vi "B7_72.vi"(4 "error in":T13, 7 "Command":T14) -> (0 "error out":T13, 3 "Response":T11)   [LabVIEW 2018]
uses:
  MOKO_LabViewLibrary/MokoLowLevel/MokoLowLovelControl/MLLC_Command.ctl
  MOKO_LabViewLibrary/MokoLowLevel/MokoLowLovelControl/MLLC_Error.ctl
  MOKO_LabViewLibrary/MokoLowLevel/MokoLowLovelControl/MLLC_Mode.ctl
  MOKO_LabViewLibrary/MokoLowLevel/MokoLowLovelControl/MLLC_Response.ctl
  MOKO_LabViewLibrary/MokoLowLevel/MokoLowLovelControl/MLLC_DriverName.ctl
  MOKO_LabViewLibrary/MokoLowLevel/MokoLowLovelControl/MLLC_ResponseInit.ctl
  MOKO_LabViewLibrary/MokoLowLevel/MokoLowLovelControl/MLLC_Request.ctl
  MOKO_LabViewLibrary/MokoLowLevel/MokoLowLovelControl/MLLC_ErrorCode.ctl
  MOKO_LabViewLibrary/MokoLowLevel/MokoLowLovelControl/MLLC_ConnectCluster.ctl
  MOKO_LabViewLibrary/MokoLowLevel/MokoLowLovelControl/MLLC_InterfaceType.ctl
  MOKO_LabViewLibrary/MokoLowLevel/MokoLowLovelControl/MLLC_OpenedSession.ctl
  MOKO_LabViewLibrary/MokoLowLevel/MokoLowLovelControl/MLLC_InterfaceSettings.ctl
  MOKO_LabViewLibrary/MokoLowLevel/MokoLowLovelControl/MLLC_InterfaceKind.ctl
  MOKO_LabViewLibrary/MokoLowLevel/MokoLowLovelControl/MLLC_Rs232Settings.ctl
panel:
  in  "Settings":T7={"Data"={"Connect"={"InterfaceType"=enum."VISA", "OpenedSession"="COM1", "InterfaceSettings"={"Interface"=enum."RS232", "EOS 4 read"=enum."LF (\\n)", "EOS 4 write"=enum."LF (\\n)", "TMO, ms"=10000, "Sett"=variant(cluster{"Baud Rate":u32, "Data Bits":u16, "Parity":u16, "Stop Bits":u16, "Flow Control":u16, "Eho":bool} {"Baud Rate"=75, "Data Bits"=0, "Parity"=0, "Stop Bits"=0, "Flow Control"=0, "Eho"=FALSE})}}, "Delay, ms"=100, "Function"=enum."VDC"}, "Saved Data"=variant}
  in  "Error Code":T6=5422
  in  "Request":T8="B2"
  in  "ResponseInit":T9="U4G1A0"
  in  "Driver Name":T10="B7_72"
  in  "Mode":T12=enum."Check"
  # "B7-72"
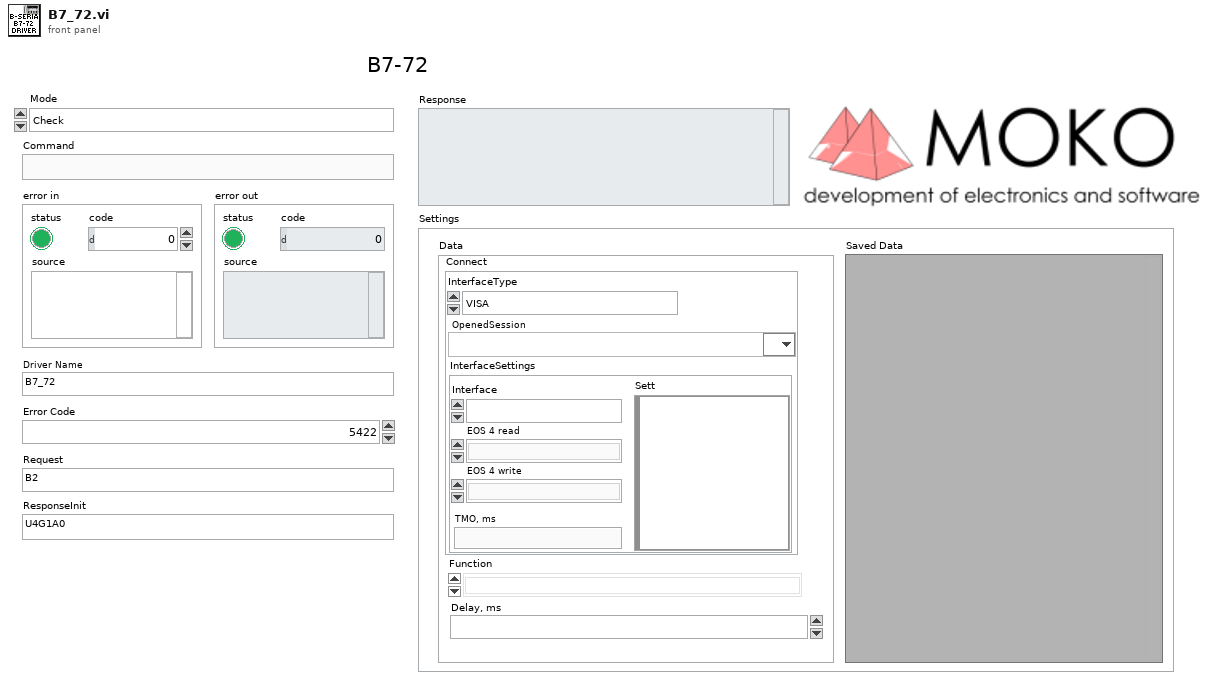
[diagram p1: front panel]
types:
  T1 = typedef "MLLC_ConnectCluster.ctl" = cluster{"InterfaceType":T2, "OpenedSession":T3, "InterfaceSettings":T4}
  T2 = typedef "MLLC_InterfaceType.ctl" = enum16{"VISA", "Prologix USB-GPIB"}
  T3 = typedef "MLLC_OpenedSession.ctl" = refnum<visa-resource-name>
  T4 = typedef "MLLC_InterfaceSettings.ctl" = cluster{"Interface":T5, "EOS 4 read":enum16{"Default (=EOS 4 write)", "CR (\\r)", "LF (\\n)", "None"}, "EOS 4 write":enum16{"CR+LF (\\r\\n)", "CR (\\r)", "LF (\\n)", "None"}, "TMO, ms":i32, "Sett":variant}
  T5 = typedef "MLLC_InterfaceKind.ctl" = enum16{"RS232", "GPIB", "USB", "Ethernet", "another"}
  T6 = typedef "MLLC_ErrorCode.ctl" = u32
  T7 = cluster{"Data":cluster{"Connect":T1, "Delay, ms":T6, "Function":enum16{"F", "T", "R4", "R", "IAC", "IDC", "VAC", "VDC"}}, "Saved Data":variant}
  T8 = typedef "MLLC_Request.ctl" = string
  T9 = typedef "MLLC_ResponseInit.ctl" = string
  T10 = typedef "MLLC_DriverName.ctl" = string
  T11 = typedef "MLLC_Response.ctl" = string
  T12 = typedef "MLLC_Mode.ctl" = enum16{"get", "set", "close", "Init", "Check"}
  T13 = typedef "MLLC_Error.ctl" = errorcluster
  T14 = typedef "MLLC_Command.ctl" = string
  T15 = cluster{"Connect":T1, "Delay, ms":T6, "Function":enum16{"F", "T", "R4", "R", "IAC", "IDC", "VAC", "VDC"}}
  T16 = enum16{"F", "T", "R4", "R", "IAC", "IDC", "VAC", "VDC"}
  T17 = typedef "MLLC_Rs232Settings.ctl" = cluster{"Baud Rate":u32, "Data Bits":u16, "Parity":u16, "Stop Bits":u16, "Flow Control":u16, "Eho":bool, "Address":dbl}
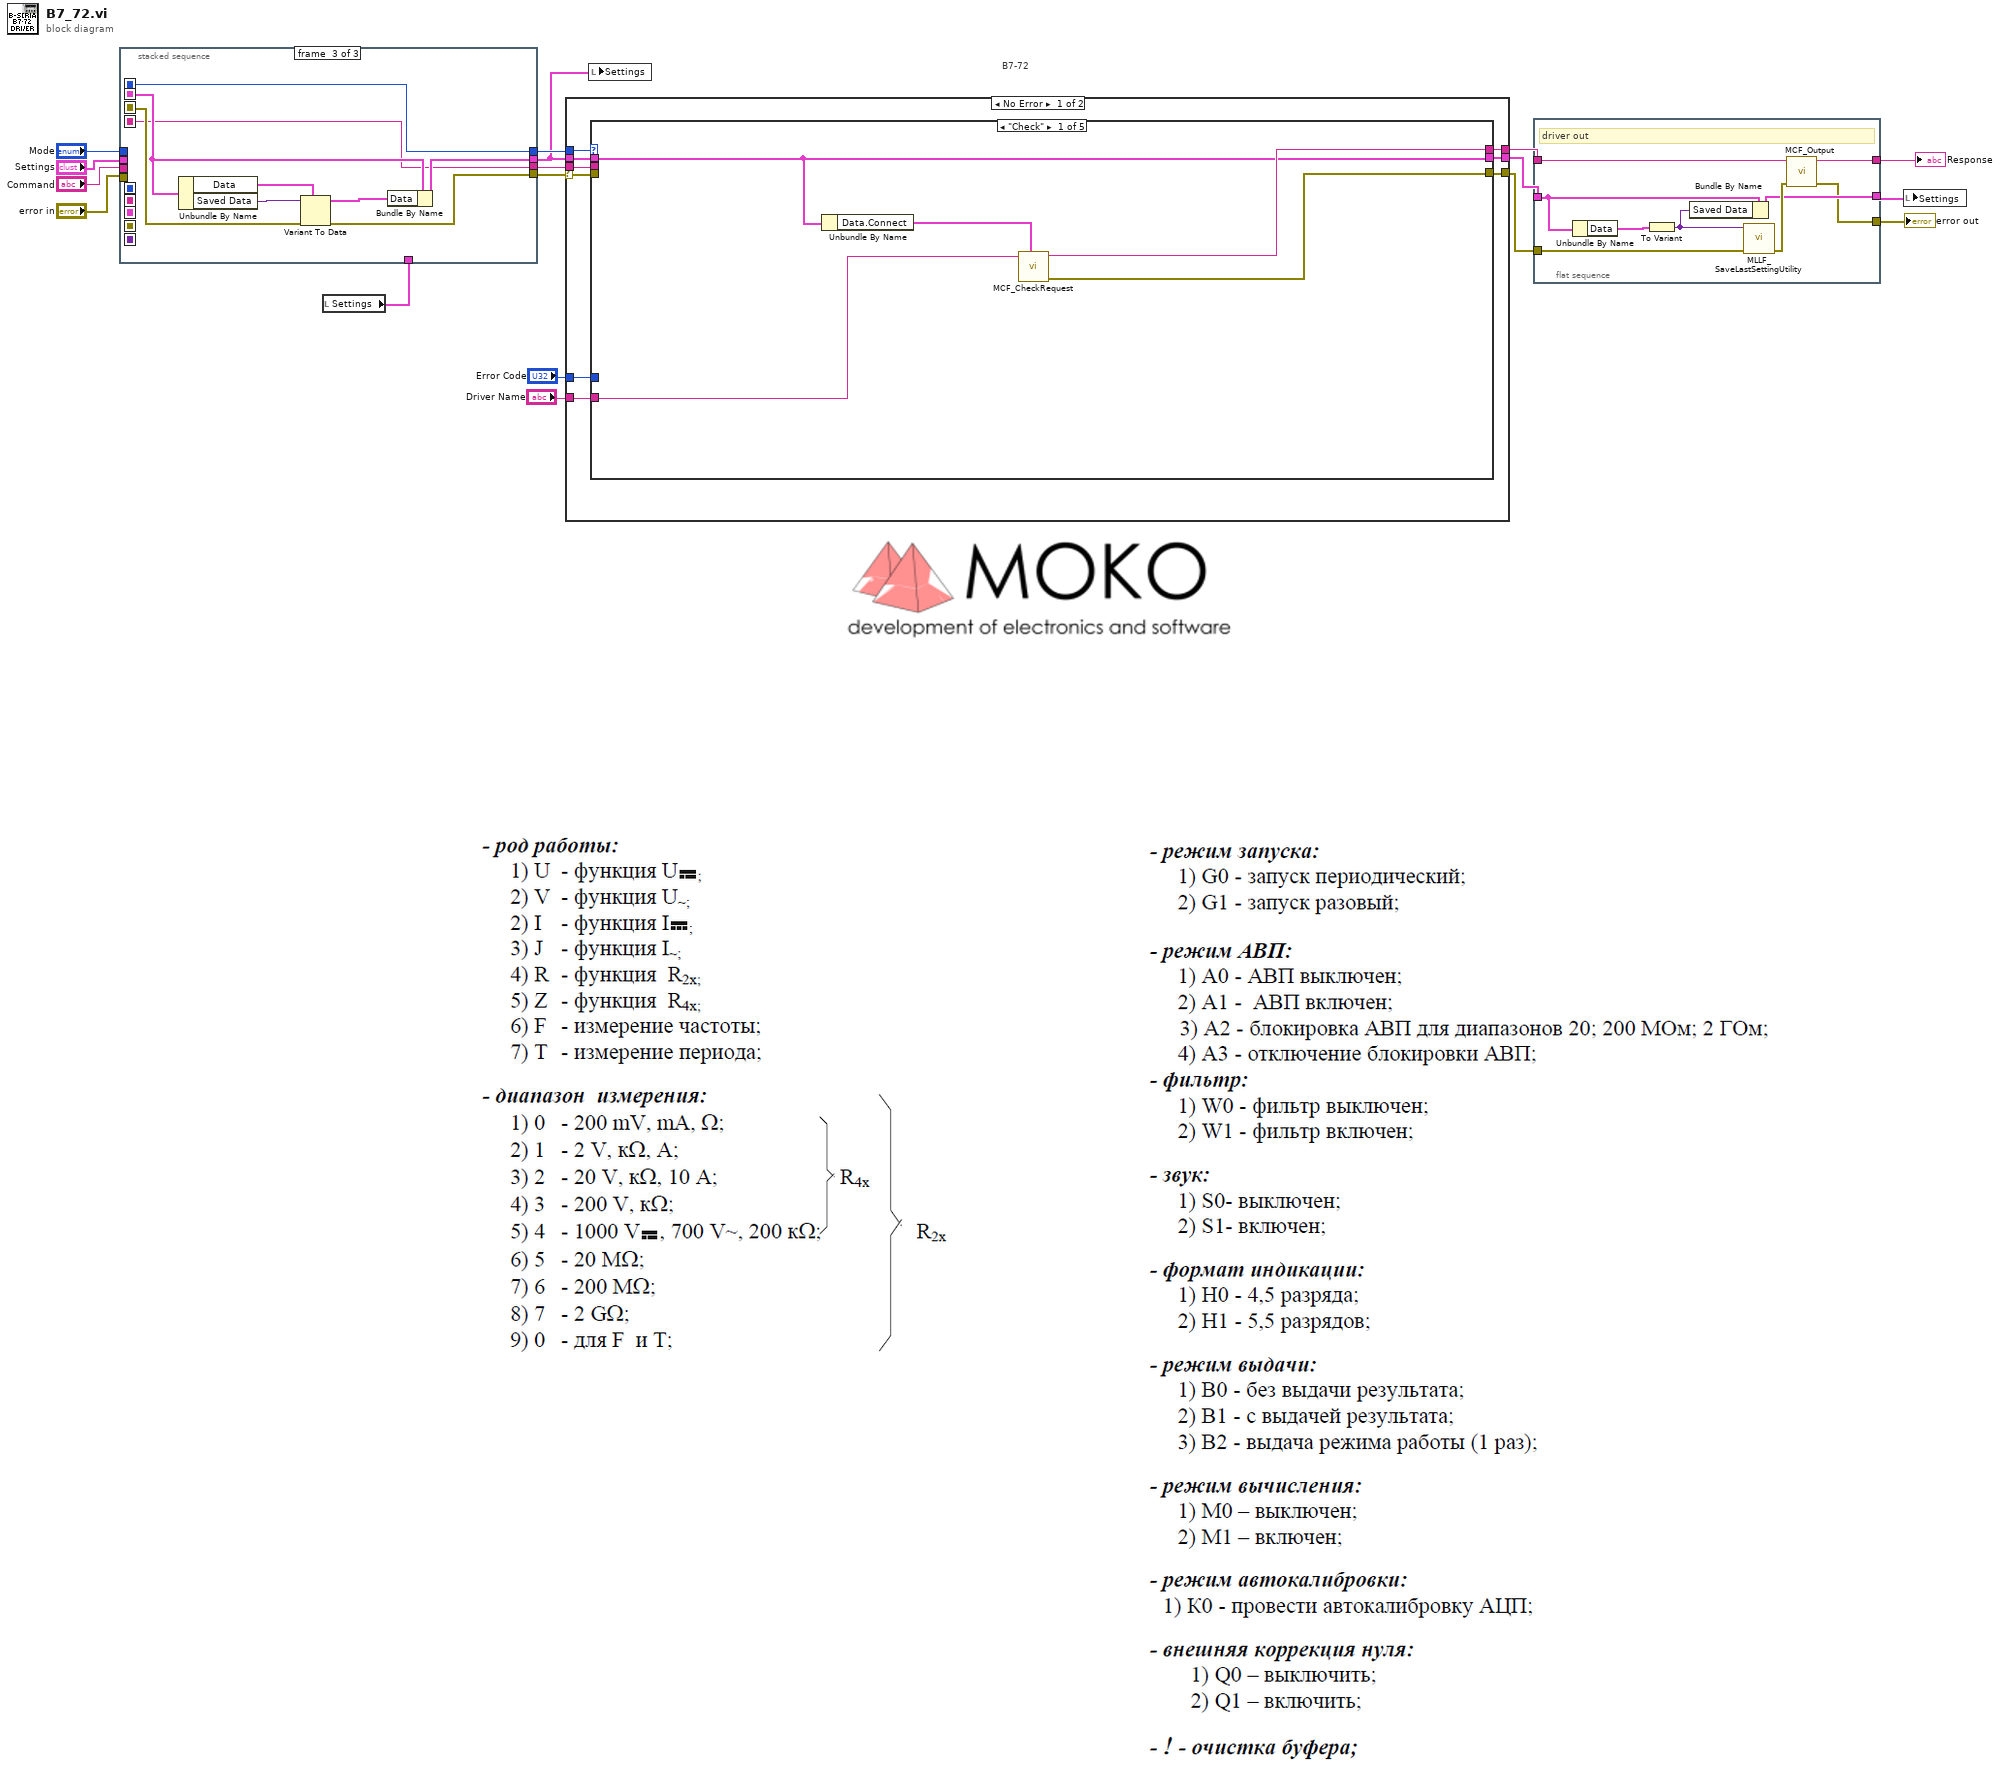
[diagram p0: block diagram]
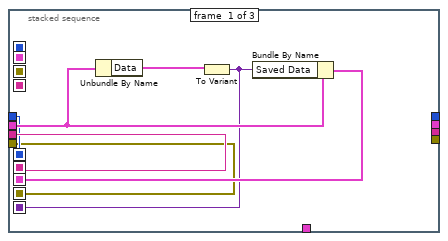
[diagram p2: hidden frame]
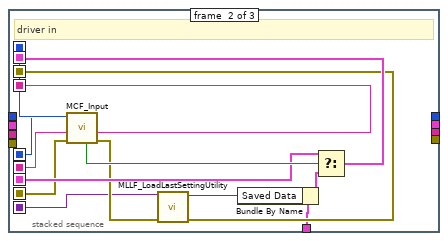
[diagram p3: hidden frame]
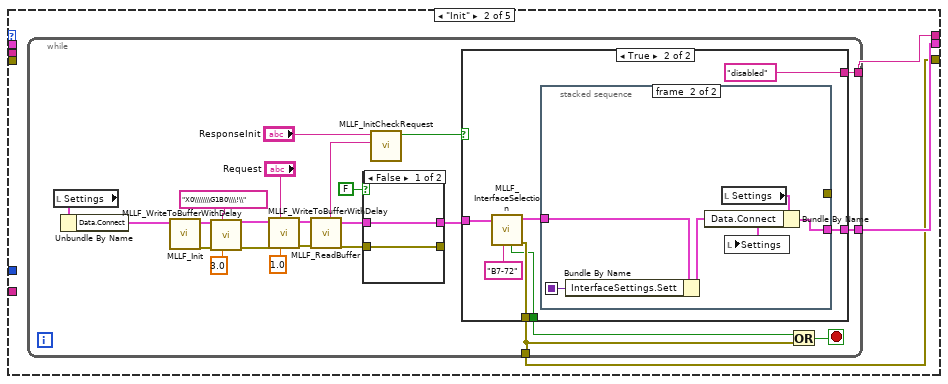
[diagram p4: hidden frame]
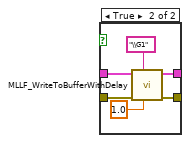
[diagram p5: hidden frame]
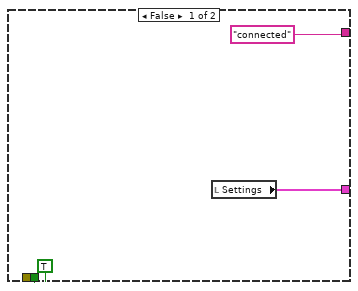
[diagram p6: hidden frame]
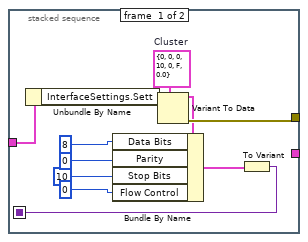
[diagram p7: hidden frame]
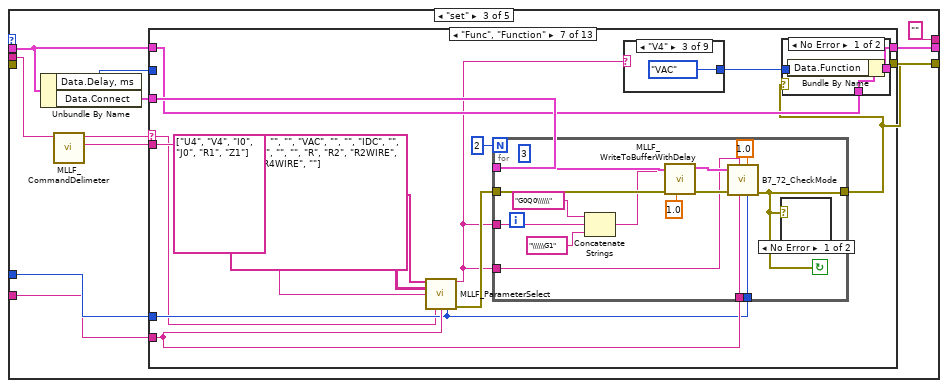
[diagram p8: hidden frame]
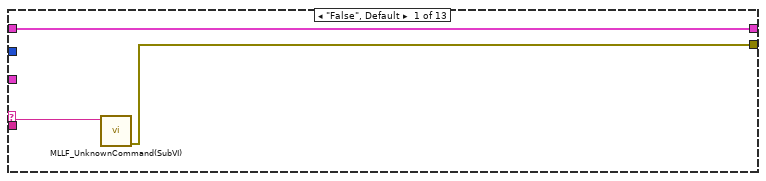
[diagram p9: hidden frame]
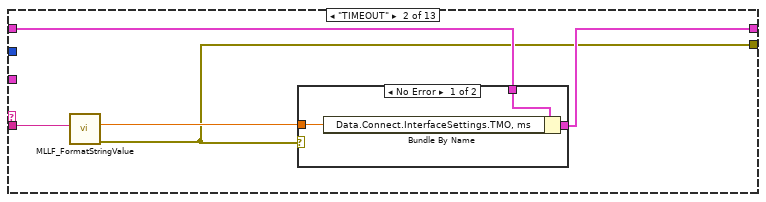
[diagram p10: hidden frame]
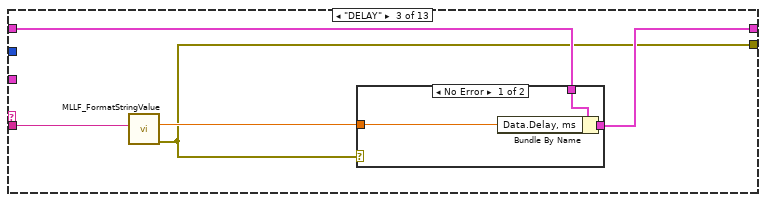
[diagram p12: hidden frame]
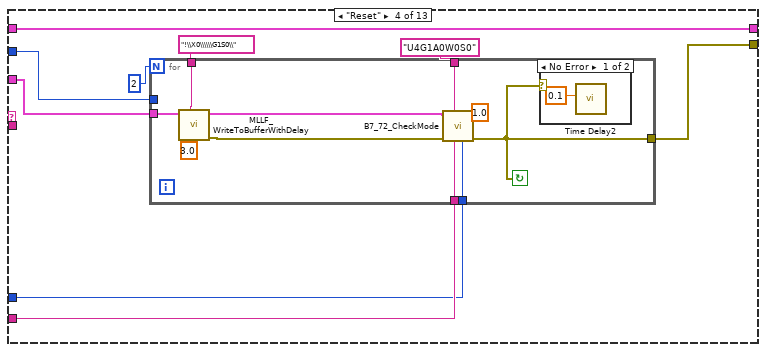
[diagram p14: hidden frame]
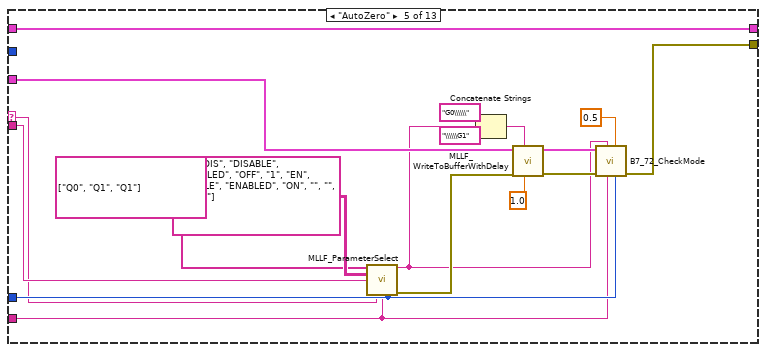
[diagram p16: hidden frame]
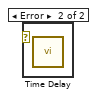
[diagram p18: hidden frame]
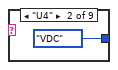
[diagram p20: hidden frame]
diagram:
  # "B7-72"
  n1 = local read "Settings"() -> (w11:T7)
  n2 = stacked-sequence {
    seq-local: [w20 _ _] -> [_ w36 _]
    seq-local: [w19 _ _] -> [_ w37 _]
    seq-local: [w22 _ _] -> [_ w32 _]
    seq-local: [w18 _ _] -> [_ w31 _]
    seq-local: [w21 _ _] -> [_ w27 _]
    seq-local: [_ w28 _] -> [_ _ w44]
    seq-local: [_ w38 _] -> [_ _ w41]
    seq-local: [_ w35 _] -> [_ _ w40]
    seq-local: [_ w34 _] -> [_ _ w45]
    tunnel: "Command" -> [w20 _ _]
    tunnel: "Mode" -> [w19 _ _]
    tunnel: "error in" -> [w18 _ _]
    tunnel: "Settings" -> [w23 _ _]
    tunnel: w11 -> [_ w26 _]
    tunnel: [_ _ w40] -> w8
    tunnel: [_ _ w43] -> w9
    tunnel: [_ _ w42] -> w7
    tunnel: [_ _ w41] -> w10
    frame #0 {
      n3 = Unbundle By Name(w23) -> ("Data"=w24:T15)
      n4 = To Variant(anything=w24) -> (Variant=w21:variant)
      n5 = Bundle By Name(cluster=w23, "Saved Data"=w21) -> (w22:T7)
    }
    frame #1 {
      # "driver in"
      n6 = call "MCF_Input.vi"("Error In"=w31, "Command in"=w36, "Mode in"=w37) -> ("Error Out"=w30:errorcluster, "Command out"=w35:string, "Mode out"=w38:T12, "Boolean"=w33:bool)  [unwired: 5 in]
      n7 = call "MLLF_LoadLastSettingUtility.vi"("Error In"=w30, "Save data in"=w27) -> ("Error Out"=w28:errorcluster, "Save data out"=w25:variant)  [unwired: 8 in]
      n8 = Bundle By Name(cluster=w26, "Saved Data"=w25) -> (w29:T7)
      n9 = Select(t=w32, s=w33, f=w29) -> (s? t:f=w34:T7)
    }
    frame #2 {
      n10 = Unbundle By Name(w45) -> ("Data"=w46:T15, "Saved Data"=w39:variant)
      n11 = Variant To Data(error in=w44, type=w46, Variant=w39) -> (data=w47:T15, error out=w42:errorcluster)
      n12 = Bundle By Name(cluster=w45, "Data"=w47) -> (w43:T7)
    }
  }
  n13 = case shown="No Error" w7 {
    selector: w7 -> [w54 w453]
    tunnel: w10 -> [w56 _]
    tunnel: w8 -> [w55 _]
    tunnel: w9 -> [w51 w452]
    tunnel: "Error Code" -> [w53 _]
    tunnel: "Driver Name" -> [w52 _]
    tunnel: [w50 "" ("String")] -> w6
    tunnel: [w49 w452] -> w5
    tunnel: [w48 w453] -> w4
    frame No Error {
      n14 = case shown="\"Check\"" w56 {
        tunnel: [w61 w64 "" ("String") w386 "" ("String")] -> w50
        tunnel: [w60 w62 w123 w385 w449] -> w48
        tunnel: w55 -> [_ _ w133 w398 _]
        tunnel: w54 -> [_ _ _ _ _]
        tunnel: w53 -> [_ _ w132 w395 _]
        tunnel: w52 -> [w59 _ w129 w394 _]
        tunnel: w51 -> [w58 _ w131 w397 w448]
        tunnel: [w58 w63 w130 w396 w448] -> w49
        frame "Check" {
          n15 = Unbundle By Name(w58) -> ("Data.Connect"=w57:T1)
          n16 = call "MCF_CheckRequest.vi"("Permanent data.Connect"=w57, "Driver Name"=w59) -> ("Error Out"=w60:errorcluster, "Output String"=w61:string)  [unwired: 8 in]
        }
        frame "Init" {
          n17 = while {
            tunnel: [w80] -> w62
            tunnel: [w66] -> w63
            tunnel: [w65] -> w64
            stop <- w79 stop-if-true
            n18 = local read "Settings"() -> (w88:T7)
            n19 = Unbundle By Name(w88) -> ("Data.Connect"=w84:T1)
            n20 = call "MLLF_Init.vi"("DriverConnect in"=w84) -> ("Error Out"=w73:errorcluster, "DriverConnect out"=w74:T1)  [unwired: 7 in]
            n21 = call "MLLF_WriteToBufferWithDelay.vi"("Delay Time ( 0,05 s)"=3.0 ("Delay Time (s)"), "Command"="X0\\\\\\\\G1B0\\\\!\\" ("String"), "Error In"=w73, "DriverConnect in"=w74) -> ("Error Out"=w77:errorcluster, "DriverConnect out"=w76:T1)  [unwired: 6 in]
            n22 = call "MLLF_WriteToBufferWithDelay.vi"("Delay Time ( 0,05 s)"=1.0 ("Delay Time (s)"), "Command"="Request", "Error In"=w77, "DriverConnect in"=w76) -> ("Error Out"=w86:errorcluster, "DriverConnect out"=w87:T1)  [unwired: 6 in]
            n23 = call "MLLF_ReadBuffer.vi"("Error In"=w86, "DriverConnect in"=w87) -> ("Error Out"=w81:errorcluster, "DriverConnect out"=w82:T1, "String"=w68:string)  [unwired: 6 in]
            n24 = case shown="False" FALSE {
              tunnel: [w89 w95] -> _
              tunnel: [w90 w94] -> w83
              tunnel: w82 -> [w90 w93]
              tunnel: w81 -> [w89 w92]
              frame False {
              }
              frame True {
                n25 = call "MLLF_WriteToBufferWithDelay.vi"("Delay Time ( 0,05 s)"=1.0 ("Delay Time (s)"), "Command"="\\G1" ("String"), "Error In"=w92, "DriverConnect in"=w93) -> ("Error Out"=w95:errorcluster, "DriverConnect out"=w94:T1)  [unwired: 6 in]
              }
            }
            n26 = call "MLLF_InitCheckRequest.vi"("Answer"=w68, "Response Init"="ResponseInit") -> ("Design"=w67:bool)  [unwired: 6 in, 3 out]
            n27 = case shown="True" w67 {
              tunnel: w83 -> [_ w106]
              tunnel: [_ w103] -> w80
              tunnel: [TRUE w100] -> w78
              tunnel: [w97 w102] -> w66
              tunnel: ["connected" "disabled"] -> w65
              frame False {
                n28 = local read "Settings"() -> (w97:T7)
              }
              frame True {
                n29 = call "MLLF_InterfaceSelection.vi"("Driver Name"="B7-72" ("String"), "DriverConnect in"=w106) -> ("error out"=w103:T13, "DriverConnect out"=w104:T1, "stop init?"=w100:bool)  [unwired: 5 in, 2 out]
                n30 = stacked-sequence {
                  seq-local: [w108 _] -> [_ w121]
                  tunnel: w104 -> [w107 w119]
                  tunnel: [w115 _] -> _
                  tunnel: [_ w120] -> w102
                  frame #0 {
                    w116 = T17 {"Baud Rate"=0, "Data Bits"=0, "Parity"=0, "Stop Bits"=10, "Flow Control"=0, "Eho"=FALSE, "Address"=0.0}  # Cluster
                    n31 = Unbundle By Name(w107) -> ("InterfaceSettings.Sett"=w117:variant)
                    n32 = Variant To Data(type=w116, Variant=w117) -> (data=w114:T17, error out=w115:errorcluster)  [unwired: 1 in]
                    n33 = Bundle By Name(cluster=w114, "Data Bits"=u16 8 ("Serial Settings:Data Bits"), "Parity"=u16 0 ("Serial Settings:Parity"), "Stop Bits"=u16 10 ("Serial Settings:Stop Bits"), "Flow Control"=u16 0 ("Serial Settings:Flow Control")) -> (w109:T17)
                    n34 = To Variant(anything=w109) -> (Variant=w108:variant)
                  }
                  frame #1 {
                    n35 = Bundle By Name(cluster=w119, "InterfaceSettings.Sett"=w121) -> (w118:T1)
                    n36 = local read "Settings"() -> (w122:T7)
                    n37 = Bundle By Name(cluster=w122, "Data.Connect"=w118) -> (w120:T7)
                    n38 = local write "Settings"(w120) -> ()
                  }
                }
              }
            }
            n39 = Or(x=w78, y=w80) -> (x .or. y?=w79:bool)
          }
        }
        frame "set" {
          n40 = Unbundle By Name(w131) -> ("Data.Delay, ms"=w126:T6, "Data.Connect"=w127:T1)
          n41 = call "MLLF_CommandDelimeter.vi"("command with param"=w133) -> ("param 1"=w124:string, "command"=w125:string)  [unwired: 6 in, 3 out]
          n42 = case shown="\"Func\", \"Function\"" w125 {
            selector: w125 -> [w135 _ _ _ w175 _ w194 _ _ w277 w306 w331 w356]
            tunnel: w124 -> [_ w139 w148 _ w187 _ w206 w234 _ w286 w315 w339 w365]
            tunnel: [w134 w137 w146 w160 w184 _ w197 w238 _ w284 w307 w332 w359] -> w123
            tunnel: w132 -> [_ _ _ w158 w189 _ w200 w240 _ w283 w308 w334 w360]
            tunnel: w131 -> [w136 w140 w149 w156 w192 w193 w199 w245 w276 w289 w317 w342 w368]
            tunnel: [w136 w141 w150 w156 w192 w193 w204 w245 w276 w289 w317 w342 w368] -> w130
            tunnel: w127 -> [_ _ _ w157 w182 _ w202 w242 _ w281 w312 w337 w363]
            tunnel: w129 -> [_ _ _ w159 w188 _ w201 w239 _ w282 w309 w333 w361]
            tunnel: w126 -> [_ _ _ w155 _ _ _ _ _ w278 _ _ w357]
            frame "False", Default {
              n43 = call "MLLF_UnknownCommand(SubVI).vi"("Unknown command"=w135) -> ("error out"=w134:errorcluster)  [unwired: 10 in]
            }
            frame "TIMEOUT" {
              n44 = call "MLLF_FormatStringValue.vi"("String Value"=w139) -> ("error out"=w137:T13, "number"=w138:dbl)  [unwired: 8 in, 1 out]
              n45 = case shown="No Error" w137 {
                tunnel: [w144 w145] -> w141
                tunnel: w140 -> [w143 w145]
                tunnel: w138 -> [w142 _]
                frame No Error {
                  n46 = Bundle By Name(cluster=w143, "Data.Connect.InterfaceSettings.TMO, ms"=w142) -> (w144:T7)
                }
                frame Error {
                }
              }
            }
            frame "DELAY" {
              n47 = call "MLLF_FormatStringValue.vi"("String Value"=w148) -> ("error out"=w146:T13, "number"=w147:dbl)  [unwired: 8 in, 1 out]
              n48 = case shown="No Error" w146 {
                tunnel: [w153 w154] -> w150
                tunnel: w149 -> [w152 w154]
                tunnel: w147 -> [w151 _]
                frame No Error {
                  n49 = Bundle By Name(cluster=w152, "Data.Delay, ms"=w151) -> (w153:T7)
                }
                frame Error {
                }
              }
            }
            frame "Reset" {
              n50 = for {
                N: 2 -> [_]
                tunnel: w157 -> [w173]
                tunnel: w159 -> [w171]
                tunnel: w158 -> [w170]
                tunnel: [w164] -> w160
                tunnel: "!\\X0\\\\\\G1S0\\" ("String") -> [w169]
                tunnel: "U4G1A0W0S0" ("Mode2check") -> [w166]
                tunnel: w155 -> [_]
                stop <- w164 continue-if-true
                n51 = call "MLLF_WriteToBufferWithDelay.vi"("Delay Time ( 0,05 s)"=3.0 ("Delay Time (s)"), "Command"=w169, "DriverConnect in"=w173) -> ("Error Out"=w165:errorcluster, "DriverConnect out"=w172:T1)  [unwired: 7 in]
                n52 = call "B7_72_CheckMode.vi"("Error Code"=w170, "Delay Time (s)"=1.0, "Driver Name"=w171, "Mode2check"=w166, "error in"=w165, "DriverConnect in"=w172) -> ("error out"=w164:T13)  [unwired: 4 in, 1 out]
                n53 = case shown="No Error" w164 {
                  frame No Error {
                    n54 = call "Time Delay2"("Delay Time (s)"=0.1) -> ()  [unwired: 10 in, 1 out]
                  }
                  frame Error {
                  }
                }
              }
            }
            frame "AutoZero" {
              n55 = call "MLLF_ParameterSelect.vi"("Command to equipment"=string[] ["Q0", "Q1", "Q1"] ("Names"), "Names"=string[][] [["0", "DIS", "DISABLE", "DISABLED", "OFF"], ["1", "EN", "ENABLE", "ENABLED", "ON"], ["", "", "", "", ""]], "Input"=w187, "Command"=w175, "Driver Name"=w188, "Error Code"=w189) -> ("Choice"=w180:string, "Error Out"=w181:errorcluster)  [unwired: 8 in]
              n56 = Concatenate Strings("G0\\\\\\" ("string"), w180, "\\\\\\G1" ("string")) -> (w179:string)
              n57 = call "MLLF_WriteToBufferWithDelay.vi"("Delay Time ( 0,05 s)"=1.0 ("Delay Time (s)"), "Command"=w179, "Error In"=w181, "DriverConnect in"=w182) -> ("Error Out"=w183:errorcluster, "DriverConnect out"=w186:T1)  [unwired: 6 in]
              n58 = call "B7_72_CheckMode.vi"("Error Code"=w189, "Delay Time (s)"=0.5, "Driver Name"=w188, "Mode2check"=w180, "error in"=w183, "DriverConnect in"=w186) -> ("error out"=w184:T13)  [unwired: 4 in, 1 out]
            }
            frame "--------------------Main----------------------" {
            }
            frame "Func", "Function" {
              n59 = call "MLLF_ParameterSelect.vi"("Command to equipment"=string[] ["U4", "V4", "I0", "J0", "R1", "Z1"] ("Names"), "Names"=string[][] [["VDC", "", ""], ["VAC", "", ""], ["IDC", "", ""], ["IAC", "", ""], ["R", "R2", "R2WIRE"], ["R4", "R4WIRE", ""]], "Input"=w206, "Command"=w194, "Driver Name"=w201, "Error Code"=w200) -> ("Choice"=w195:string, "Error Out"=w198:errorcluster)  [unwired: 8 in]
              n60 = for {
                N: 2 -> [_]
                tunnel: w202 -> [w221]
                tunnel: w201 -> [w217]
                tunnel: w200 -> [w216]
                tunnel: w198 -> [w220]
                tunnel: [w214] -> w197
                tunnel: w195 -> [w212]
                tunnel: w195 -> [w213]
                stop <- w214 continue-if-true
                (unwired) 3
                n61 = Concatenate Strings("G0Q0\\\\\\" ("string"), w213, "\\\\\\G1" ("string")) -> (w210:string)
                n62 = call "MLLF_WriteToBufferWithDelay.vi"("Delay Time ( 0,05 s)"=1.0 ("Delay Time (s)"), "Command"=w210, "Error In"=w220, "DriverConnect in"=w221) -> ("Error Out"=w215:errorcluster, "DriverConnect out"=w219:T1)  [unwired: 6 in]
                n63 = call "B7_72_CheckMode.vi"("Error Code"=w216, "Delay Time (s)"=1.0, "Driver Name"=w217, "Mode2check"=w212, "error in"=w215, "DriverConnect in"=w219) -> ("error out"=w214:T13)  [unwired: 4 in, 1 out]
                n64 = case shown="No Error" w214 {
                  frame No Error {
                  }
                  frame Error {
                    n65 = call "Time Delay"() -> ()  [unwired: 11 in, 1 out]
                  }
                }
              }
              n66 = case shown="\"V4\"" w195 {
                tunnel: [_ T16."VDC" ("Function") T16."VAC" ("Function") T16."IDC" ("Function") T16."IAC" ("Function") T16."R" ("Function") T16."R4" ("Function") T16."F" ("Function") T16."T" ("Function")] -> w203
                frame "False", Default {
                }
                frame "U4" {
                }
                frame "V4" {
                }
                frame "I0" {
                }
                frame "J0" {
                }
                frame "R1" {
                }
                frame "Z1" {
                }
                frame "F0" {
                }
                frame "T0" {
                }
              }
              n67 = case shown="No Error" w197 {
                tunnel: [w232 w233] -> w204
                tunnel: w199 -> [w231 w233]
                tunnel: w203 -> [w230 _]
                frame No Error {
                  n68 = Bundle By Name(cluster=w231, "Data.Function"=w230) -> (w232:T7)
                }
                frame Error {
                }
              }
            }
            frame "RANGE" {
              n69 = Unbundle By Name(w245) -> ("Data.Function"=w246:T16)
              n70 = Index Array(array=string[] ["F", "T", "Z", "R", "J", "I", "V", "U"] ("Names"), index=w246) -> (element=w244:string)
              n71 = case shown="\"1\", Default" w234 {
                selector: w234 -> [w260 _]
                tunnel: [w261 _] -> w241
                tunnel: [w264 "1A1" ("String")] -> w243
                tunnel: w244 -> [w265 _]
                frame "1", Default {
                  n72 = call "MLLF_FormatStringValue.vi"("String Value"=w260) -> ("error out"=w261:T13, "number"=w263:dbl)  [unwired: 8 in, 1 out]
                  n73 = case shown="\"R\", \"Z\"" w265 {
                    tunnel: [w266 w273 "0" ("R/O")] -> w264
                    tunnel: w263 -> [w267 w270 _]
                    tunnel: string[] ["0", "1", "2", "3", "4", "5", "6", "7"] ("RangeCommand") -> [w269 w272 _]
                    frame "R", "Z" {
                      n74 = call "B7_72_82_StandartRangeSelect (SubVI).vi"("Control Point"=w267, "RangeDigit"=dbl[] [200.0, 2000.0, 20000.0, 200000.0, 2000000.0, 20000000.0, 200000000.0, 2000000000.0], "RangeCommand"=w269) -> ("R/O"=w266:string)  [unwired: 1 in]
                    }
                    frame "U", "V", Default {
                      n75 = call "B7_72_82_StandartRangeSelect (SubVI).vi"("Control Point"=w270, "RangeDigit"=dbl[] [0.2, 2.0, 20.0, 200.0, 1000.0], "RangeCommand"=w272) -> ("R/O"=w273:string)  [unwired: 1 in]
                    }
                    frame "I", "J" {
                    }
                  }
                }
                frame "auto" {
                }
              }
              n76 = Concatenate Strings(w244, w243) -> (w237:string)
              n77 = for {
                N: 2 -> [_]
                tunnel: w242 -> [w252]
                tunnel: w239 -> [w258]
                tunnel: w240 -> [w257]
                tunnel: w241 -> [w253]
                tunnel: [w256] -> w238
                tunnel: w237 -> [w249]
                stop <- w256 continue-if-true
                n78 = Concatenate Strings("G0Q0\\\\\\" ("string"), w249, "\\\\\\G1" ("string")) -> (w250:string)
                n79 = call "MLLF_WriteToBufferWithDelay.vi"("Delay Time ( 0,05 s)"=1.0 ("Delay Time (s)"), "Command"=w250, "Error In"=w253, "DriverConnect in"=w252) -> ("Error Out"=w254:errorcluster, "DriverConnect out"=w255:T1)  [unwired: 6 in]
                n80 = call "B7_72_CheckMode.vi"("Error Code"=w257, "Delay Time (s)"=0.5, "Driver Name"=w258, "Mode2check"=w249, "error in"=w254, "DriverConnect in"=w255) -> ("error out"=w256:T13)  [unwired: 4 in, 1 out]
                n81 = case shown="Error" w256 {
                  frame No Error {
                  }
                  frame Error {
                    n82 = call "Time Delay6"() -> ()  [unwired: 11 in, 1 out]
                  }
                }
              }
            }
            frame "-------------Supplemental------------" {
            }
            frame "ACQ", "ACQUISITION" {
              # "В этой функции большого смысла нет!"
              n83 = call "MLLF_ParameterSelect.vi"("Command to equipment"=string[] ["G0", "G1"] ("Names"), "Names"=string[][] [["CONT", "CONTINUOUS", ""], ["ONCE", "ONETIME", "1"]], "Input"=w286, "Command"=w277, "Driver Name"=w282, "Error Code"=w283) -> ("Choice"=w280:string, "Error Out"=w279:errorcluster)  [unwired: 8 in]
              n84 = for {
                N: 2 -> [_]
                tunnel: w281 -> [w305]
                tunnel: w283 -> [w303]
                tunnel: w282 -> [w302]
                tunnel: [w299] -> w284
                tunnel: w279 -> [w300]
                tunnel: w280 -> [w290]
                tunnel: w278 -> [w292]
                stop <- w299 continue-if-true
                n85 = Concatenate Strings(w290) -> (w291:string)
                n86 = call "MLLF_WriteToBufferWithDelay.vi"("Delay Time ( 0,05 s)"=3.0 ("Delay Time (s)"), "Command"=w291, "Error In"=w300, "DriverConnect in"=w305) -> ("Error Out"=w293:errorcluster, "DriverConnect out"=w304:T1)  [unwired: 6 in]
                n87 = Divide(x=w292, y=1000) -> (x/y=w295:dbl)
                n88 = call "Time Delay5"("error in (no error)"=w293, "Delay Time (s)"=w295) -> ("error out"=w294:errorcluster)  [unwired: 9 in]
                n89 = Wait (ms)(milliseconds to wait=u32 100) -> ()  [unwired: 1 out]
                n90 = call "B7_72_CheckMode.vi"("Error Code"=w303, "Delay Time (s)"=0.5, "Driver Name"=w302, "Mode2check"=w290, "error in"=w294, "DriverConnect in"=w304) -> ("error out"=w299:T13)  [unwired: 4 in, 1 out]
              }
            }
            frame "Filter" {
              n91 = call "MLLF_ParameterSelect.vi"("Command to equipment"=string[] ["W0", "W1"] ("Names"), "Names"=string[][] [["0", "DIS", "DISABLED", "DISABLE", "OFF"], ["1", "EN", "ENABLE", "ENABLED", "ON"]], "Input"=w315, "Command"=w306, "Driver Name"=w309, "Error Code"=w308) -> ("Choice"=w310:string, "Error Out"=w311:errorcluster)  [unwired: 8 in]
              n92 = for {
                N: 2 -> [_]
                tunnel: w312 -> [w330]
                tunnel: w309 -> [w325]
                tunnel: w308 -> [w324]
                tunnel: [w322] -> w307
                tunnel: w311 -> [w319]
                tunnel: w310 -> [w318]
                stop <- w322 continue-if-true
                n93 = Concatenate Strings("G0Q0\\" ("string"), w318, "\\\\G1" ("string")) -> (w329:string)
                n94 = call "MLLF_WriteToBufferWithDelay.vi"("Delay Time ( 0,05 s)"=1.0 ("Delay Time (s)"), "Command"=w329, "Error In"=w319, "DriverConnect in"=w330) -> ("Error Out"=w323:errorcluster, "DriverConnect out"=w328:T1)  [unwired: 6 in]
                n95 = call "B7_72_CheckMode.vi"("Error Code"=w324, "Delay Time (s)"=0.5, "Driver Name"=w325, "Mode2check"=w318, "error in"=w323, "DriverConnect in"=w328) -> ("error out"=w322:T13)  [unwired: 4 in, 1 out]
                n96 = case shown="Error" w322 {
                  frame No Error {
                  }
                  frame Error {
                    n97 = call "Time Delay3"() -> ()  [unwired: 11 in, 1 out]
                  }
                }
              }
            }
            frame "DIGITS", "DISP", "DISPLAY", "INTEGRATIONTIME", "INTTIME" {
              n98 = call "MLLF_ParameterSelect.vi"("Command to equipment"=string[] ["H1", "H0"] ("Names"), "Names"=string[][] [["6.5", "6,5", "7"], ["5.5", "5,5", "6"]], "Input"=w339, "Command"=w331, "Driver Name"=w333, "Error Code"=w334) -> ("Choice"=w335:string, "Error Out"=w336:errorcluster)  [unwired: 8 in]
              n99 = for {
                N: 2 -> [_]
                tunnel: w337 -> [w355]
                tunnel: w333 -> [w350]
                tunnel: w334 -> [w349]
                tunnel: [w347] -> w332
                tunnel: w336 -> [w344]
                tunnel: w335 -> [w343]
                stop <- w347 continue-if-true
                n100 = Concatenate Strings("G0Q0\\" ("string"), w343, "\\\\G1" ("string")) -> (w354:string)
                n101 = call "MLLF_WriteToBufferWithDelay.vi"("Delay Time ( 0,05 s)"=1.0 ("Delay Time (s)"), "Command"=w354, "Error In"=w344, "DriverConnect in"=w355) -> ("Error Out"=w348:errorcluster, "DriverConnect out"=w353:T1)  [unwired: 6 in]
                n102 = call "B7_72_CheckMode.vi"("Error Code"=w349, "Delay Time (s)"=0.5, "Driver Name"=w350, "Mode2check"=w343, "error in"=w348, "DriverConnect in"=w353) -> ("error out"=w347:T13)  [unwired: 4 in, 1 out]
                n103 = case shown="Error" w347 {
                  frame No Error {
                  }
                  frame Error {
                    n104 = call "Time Delay4"() -> ()  [unwired: 11 in, 1 out]
                  }
                }
              }
            }
            frame "SND", "SOUND" {
              n105 = call "MLLF_ParameterSelect.vi"("Command to equipment"=string[] ["S0", "S1"] ("Names"), "Names"=string[][] [["0", "DIS", "DISABLED", "DISABLE", "OFF"], ["1", "EN", "ENABLE", "ENABLED", "ON"]], "Input"=w365, "Command"=w356, "Driver Name"=w361, "Error Code"=w360) -> ("Choice"=w362:string, "Error Out"=w358:errorcluster)  [unwired: 8 in]
              n106 = for {
                N: 2 -> [_]
                tunnel: w363 -> [w384]
                tunnel: w360 -> [w382]
                tunnel: w361 -> [w381]
                tunnel: [w379] -> w359
                tunnel: w362 -> [w369]
                tunnel: w358 -> [w378]
                tunnel: w357 -> [w373]
                stop <- w379 continue-if-true
                n107 = Concatenate Strings(w369) -> (w370:string)
                n108 = call "MLLF_WriteToBufferWithDelay.vi"("Delay Time ( 0,05 s)"=2.0 ("Delay Time (s)"), "Command"=w370, "Error In"=w378, "DriverConnect in"=w384) -> ("Error Out"=w374:errorcluster, "DriverConnect out"=w383:T1)  [unwired: 6 in]
                n109 = Divide(x=w373, y=1000) -> (x/y=w372:dbl)
                n110 = call "Time Delay8"("error in (no error)"=w374, "Delay Time (s)"=w372) -> ("error out"=w375:errorcluster)  [unwired: 9 in]
                n111 = Wait (ms)(milliseconds to wait=u32 100) -> ()  [unwired: 1 out]
                n112 = call "B7_72_CheckMode.vi"("Error Code"=w382, "Delay Time (s)"=0.5, "Driver Name"=w381, "Mode2check"=w369, "error in"=w375, "DriverConnect in"=w383) -> ("error out"=w379:T13)  [unwired: 4 in, 1 out]
              }
            }
          }
        }
        frame "get" {
          n113 = Unbundle By Name(w397) -> ("Data.Connect"=w391:T1, "Data.Function"=w389:T16)
          n114 = call "MLLF_CommandDelimeter.vi"("command with param"=w398) -> ("param 1"=w387:string, "command"=w388:string)  [unwired: 6 in, 3 out]
          n115 = case shown="\"TIMEOUT\"" w388 {
            selector: w388 -> [w400 _ _]
            tunnel: [w399 _ w409] -> w393
            tunnel: w395 -> [_ _ _]
            tunnel: [w403 w406 w413] -> w396
            tunnel: w397 -> [w403 w406 w413]
            tunnel: [w401 w404 w410] -> w392
            tunnel: w391 -> [_ _ w411]
            tunnel: w394 -> [_ _ _]
            tunnel: w387 -> [_ _ w412]
            tunnel: w389 -> [_ _ w407]
            frame "False", Default {
              n116 = call "MLLF_UnknownCommand(SubVI).vi"("Unknown command"=w400) -> ("error out"=w399:errorcluster)  [unwired: 10 in]
              n117 = Build Array(0 ("TimeOut")) -> (w401:i32[])
            }
            frame "TIMEOUT" {
              n118 = Unbundle By Name(w406) -> ("Data.Connect.InterfaceSettings.TMO, ms"=w405:i32)
              n119 = Build Array(w405) -> (w404:i32[])
            }
            frame "FETCH", "READ" {
              n120 = for {
                N: 3 -> [_]
                tunnel: w412 -> [w439]
                tunnel: w411 -> [w420]
                tunnel: [w414] -> w410
                tunnel: [w427] -> w409
                tunnel: w407 -> [_]
                stop <- w427 continue-if-true
                n121 = Decimal String To Number(string=w439) -> (number=w438:i32)  [unwired: 2 in, 1 out]
                n122 = call "MLLF_WriteToBufferWithDelay.vi"("Delay Time ( 0,05 s)"=2.0 ("Delay Time (s)"), "Command"="G0B1\\\\\\!" ("String"), "DriverConnect in"=w420) -> ("Error Out"=w424:errorcluster, "DriverConnect out"=w425:T1)  [unwired: 7 in]
                n123 = In Range and Coerce(upper limit=100, x=w438, lower limit=1) -> (coerced(x)=w419:i32)  [unwired: 1 out]
                n124 = call "MLLF_ClearBuffer.vi"("Timeout(default = 300 ms)"=u32 500 ("Timeout"), "Error In"=w424, "DriverConnect in"=w425) -> ("Error Out"=w421:errorcluster, "DriverConnect out"=w422:T1)  [unwired: 5 in, 1 out]
                n125 = Increment(x=w419) -> (x+1=w418:i32)
                n126 = for {
                  N: w418 -> [_]
                  tunnel: [w445] -> w415 mode=indexing
                  tunnel: [w444] -> w434
                  tunnel: [w442] -> w433
                  tunnel: w422 -> [w441]
                  tunnel: w421 -> [w440]
                  stop <- w444 stop-if-true
                  n127 = call "MLLF_ReadBuffer.vi"("Error In"=w440, "DriverConnect in"=w441) -> ("Error Out"=w444:errorcluster, "DriverConnect out"=w442:T1, "String"=w443:string)  [unwired: 6 in]
                  n128 = Fract/Exp String To Number(use system decimal point (T)=FALSE, string=w443) -> (number=w445:dbl)  [unwired: 2 in, 1 out]
                }
                n129 = call "MLLF_WriteToBufferWithDelay.vi"("Delay Time ( 0,05 s)"=0.5 ("Delay Time (s)"), "Command"="\\G1B0\\!" ("String"), "Error In"=w434, "DriverConnect in"=w433) -> ("Error Out"=w428:errorcluster, "DriverConnect out"=w429:T1)  [unwired: 6 in]
                n130 = Delete From Array(array=w415, length=1, index=0) -> (array with subset deleted=w414:dbl[])  [unwired: 1 out]
                n131 = call "MLLF_ClearBuffer.vi"("Timeout(default = 300 ms)"=u32 300 ("Timeout"), "Error In"=w428, "DriverConnect in"=w429) -> ("Error Out"=w427:errorcluster)  [unwired: 5 in, 2 out]
              }
            }
          }
          n132 = call "MLLF_FormatOutputValueWithUnits.vi"("Format"="%.;%^#_7e" ("format string"), "error in"=w393, "ValuesIn"=w392) -> ("error out"=w385:T13, "Result string"=w386:T14)  [unwired: 7 in]
        }
        frame "close" {
          n133 = Unbundle By Name(w448) -> ("Data.Connect.OpenedSession"=w450:T3)
          n134 = VISA Close(VISA resource name=w450) -> (error out=w449:errorcluster)  [unwired: 1 in]
        }
      }
    }
    frame Error {
    }
  }
  n135 = local write "Settings"(w9) -> ()
  n136 = flat-sequence {
    tunnel: [w462] -> w3
    tunnel: [w454] -> _
    tunnel: w6 -> [w461]
    tunnel: w4 -> [w460]
    tunnel: w5 -> [w456]
    tunnel: [w458] -> w2
    tunnel: [w454] -> w1
    frame #0 {
      # "driver out"
      n137 = Unbundle By Name(w456) -> ("Data"=w455:T15)
      n138 = To Variant(anything=w455) -> (Variant=w457:variant)
      n139 = Bundle By Name(cluster=w456, "Saved Data"=w457) -> (w458:T7)
      n140 = call "MLLF_SaveLastSettingUtility.vi"("error in"=w460, "Saved Data"=w457) -> ("error out"=w459:T13)  [unwired: 8 in, 1 out]
      n141 = call "MCF_Output.vi"("Error In"=w459, "Input"=w461) -> ("Error Out"=w454:errorcluster, "Output"=w462:string)  [unwired: 8 in]
    }
  }
  n142 = local write "Settings"(w2) -> ()
  "error out" <- w1
  "Response" <- w3
